vi "Cartesian Displacements Offsets Dataset.vi"(7 "LBCB Number":T2, 8 "error in (no error)":errorcluster, 10 "Offsets In":T1, 11 "DAO Actions":T3) -> (0 "error out":errorcluster, 2 "Offsets Out":T1)   [LabVIEW 2009]
uses:
  Data Access Objects/Metadata/DAO Actions.ctl
  Data Access Objects/Metadata/LBCB Number.ctl
  Data Access Objects/Metadata/Cartesian Point.ctl
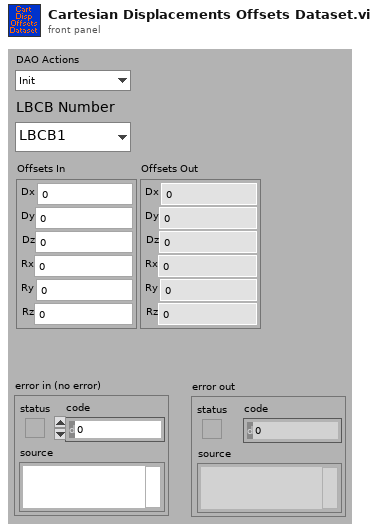
[diagram p1: front panel]
types:
  T1 = typedef "Cartesian Point.ctl" = cluster{"Dx":dbl, "Dy":dbl, "Dz":dbl, "Rx":dbl, "Ry":dbl, "Rz":dbl}
  T2 = typedef "LBCB Number.ctl" = enum16{"LBCB1", "LBCB2"}
  T3 = typedef "DAO Actions.ctl" = enum16{"Init", "Get", "Set"}
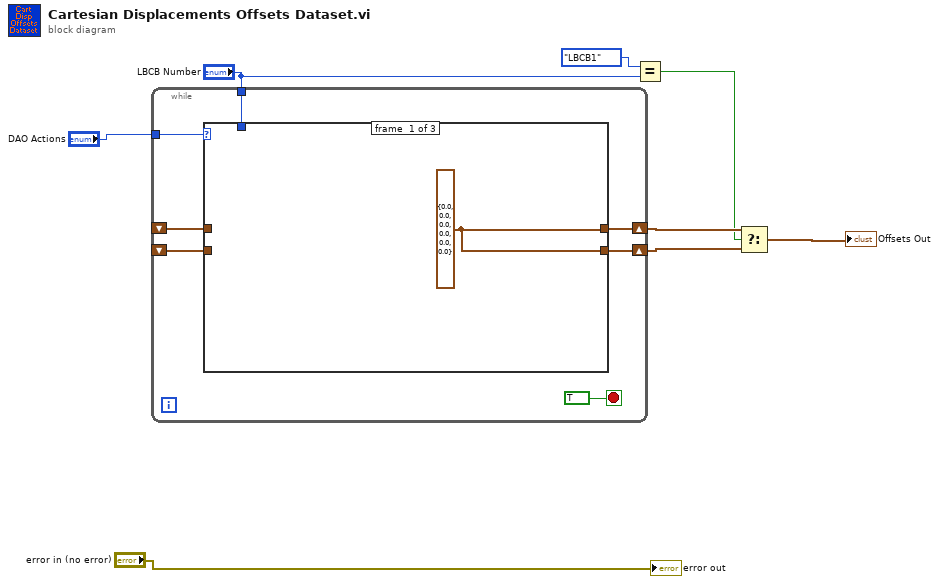
[diagram p0: block diagram]
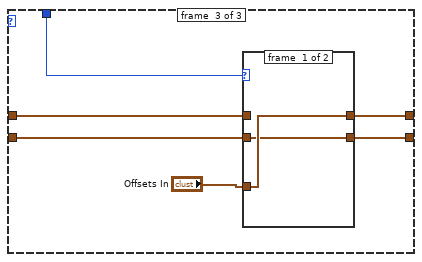
[diagram p3: hidden frame]
diagram:
  n1 = while {
    tunnel: "DAO Actions" -> [w14]
    shift-right: [w13] -> w5
    shift-left: _ -> [w10]
    tunnel: "LBCB Number" -> [w12]
    shift-right: [w11] -> w4
    shift-left: _ -> [w9]
    stop <- TRUE stop-if-true
    n2 = case shown="\"Init\"" w14 {
      tunnel: [w16 w18 w20] -> w13
      tunnel: w12 -> [_ _ w24]
      tunnel: [w16 w17 w22] -> w11
      tunnel: w10 -> [_ w18 w21]
      tunnel: w9 -> [_ w17 w19]
      frame #0 {
        w16 = T1 {"Dx"=0.0, "Dy"=0.0, "Dz"=0.0, "Rx"=0.0, "Ry"=0.0, "Rz"=0.0} ("Offsets In")
      }
      frame #1 {
      }
      frame #2 {
        n3 = case shown="\"LBCB1\"" w24 {
          tunnel: "Offsets In" -> [w26 w28]
          tunnel: [w25 w28] -> w22
          tunnel: w21 -> [_ w27]
          tunnel: [w26 w27] -> w20
          tunnel: w19 -> [w25 _]
          frame #0 {
          }
          frame #1 {
          }
        }
      }
    }
  }
  n4 = Equal?(x=LBCB_Number."LBCB1", y="LBCB Number") -> (x = y?=w1:bool)
  n5 = Select(t=w5, s=w1, f=w4) -> (s? t:f=→"Offsets Out":T1)
  "error out" <- "error in (no error)"
